vi "Get Property Enum Values.vi"(0 "SLSC Remote in":refnum<class "SLSC Remote.lvclass">, 5 "property":refnum<k21>, 11 "error in (no error)":errorcluster) -> (4 "SLSC Remote out":refnum<class "SLSC Remote.lvclass">, 6 "property out":refnum<k21>, 10 "Prop.Enum.Values":i32[](array[numeric]), 15 "error out":errorcluster)   [LabVIEW 2016, in "SLSC Interfaces.lvlib" / "SLSC Remote.lvclass"]
uses:
  SLSC Remote.lvclass
  C:/Users/tblair/Documents/Git Projects/SLSC-Interface/Source/SLSC Interface Class/SLSC Interface.lvclass
  <vilib>/National Instruments/JSON Support for LabVIEW/JSON Data Classes/JSON Object/JSON Object.lvclass
  C:/Program Files (x86)/National Instruments/LabVIEW 2016/vi.lib/National Instruments/JSON Support for LabVIEW/JSON Data Classes/JSON Datatype/JSON Datatype.lvclass
  <vilib>/National Instruments/JSON Support for LabVIEW/JSON Data Classes/JSON Object/New JSON Object (Empty).vi
  <vilib>/National Instruments/JSON Support for LabVIEW/JSON Data Classes/JSON Object/Insert Key Value Pair (Single String).vi
  <vilib>/NI/NI JSONRPC Server Framework/Classes/Server/Format Client Request (Auto-Increment).vi
  <vilib>/httpClient/POSTBuffer.vi
  <vilib>/National Instruments/JSON Support for LabVIEW/JSON Data Classes/JSON Datatype/To More Specific Type (Object).vi
  <vilib>/National Instruments/JSON Support for LabVIEW/JSON Data Classes/JSON Object/Get Value (Array).vi
  <vilib>/National Instruments/JSON Support for LabVIEW/JSON Data Classes/JSON Array/Index Array (Numeric Value).vi
  <vilib>/NI/NI JSONRPC Server Framework/Classes/Server/JSONRPC Server.lvclass
  <vilib>/httpClient/LabVIEWHTTPClient.lvlib
  <vilib>/National Instruments/JSON Support for LabVIEW/JSON Data Classes/JSON Datatype/JSON Datatype.lvclass
  <vilib>/National Instruments/JSON Support for LabVIEW/JSON Data Classes/JSON Array/JSON Array.lvclass
  C:/Program Files (x86)/National Instruments/LabVIEW 2016/vi.lib/National Instruments/JSON Support for LabVIEW/JSON Data Classes/JSON Structured Type/JSON Structured Type.lvclass
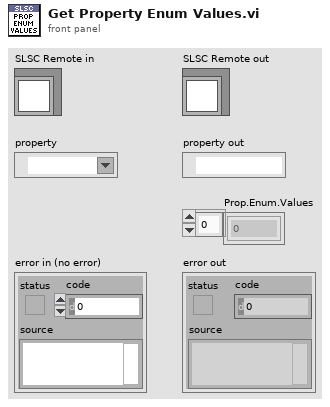
[diagram p1: front panel]
types:
  T1 = typedef "LabVIEWHTTPClient.lvlib/ClientHandle.ctl" = refnum<k1>
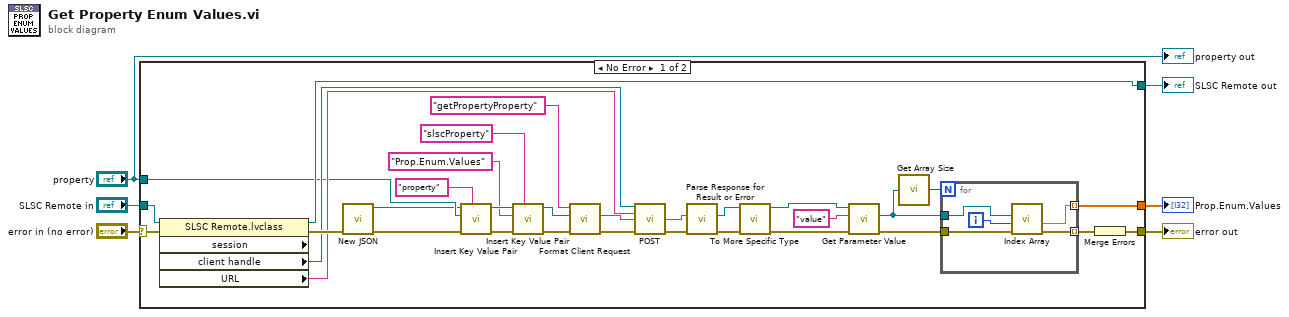
[diagram p0: block diagram]
diagram:
  n1 = case shown="No Error" "error in (no error)" {
    selector: "error in (no error)" -> [w36 w44]
    tunnel: "SLSC Remote in" -> [w38 w45]
    tunnel: [w37 w45] -> w4
    tunnel: [w13 w44] -> w2
    tunnel: "property" -> [w12 _]
    tunnel: [w14 _] -> w1
    frame No Error {
      n2 = property class="SLSC Remote.lvclass" props=["session", "client handle", "URL"](reference=w38, error in=w36) -> (reference out=w37:refnum<class "SLSC Remote.lvclass">, error out=w35:errorcluster, "client handle"=w31:T1, "URL"=w30:string)  [unwired: 1 out]
      n3 = call-poly <vilib>:"New JSON.vi"("error in (no error)"=w35) -> ("error out"=w34:errorcluster, "JSON Object out"=w9:refnum<class "JSON Object.lvclass">)  [unwired: 9 in]
      n4 = call-poly <vilib>:"Insert Key Value Pair.vi"("key"="property" ("Name"), "error in (no error)"=w34, "value"=w12, "JSON Object in"=w9) -> ("error out"=w24:errorcluster, "JSON Object out"=w10:refnum<class "JSON Object.lvclass">)  [unwired: 5 in, 1 out]
      n5 = call-poly <vilib>:"Insert Key Value Pair.vi"("key"="slscProperty" ("Name"), "error in (no error)"=w24, "value"="Prop.Enum.Values" ("String"), "JSON Object in"=w10) -> ("error out"=w25:errorcluster, "JSON Object out"=w26:refnum<class "JSON Object.lvclass">)  [unwired: 5 in, 1 out]
      n6 = call-poly <vilib>:"Format Client Request.vi"("error in (no error)"=w25, "JSON in"=w26, "method"="getPropertyProperty") -> ("error out"=w29:errorcluster, "Request String"=w32:string)  [unwired: 7 in]
      n7 = call-poly <vilib>:"POST.vi"("client handle"=w31, "url"=w30, "buffer"=w32, "error in (no error)"=w29) -> ("body"=w28:string, "error out"=w27:errorcluster)  [unwired: 8 in, 2 out]
      n8 = call <vilib>:"Parse Response for Result or Error.vi"("error in"=w27, "Response String In"=w28) -> ("error out"=w16:errorcluster, "JSON out"=w17:refnum<class "JSON Datatype.lvclass">)  [unwired: 7 in, 1 out]
      n9 = call-poly <vilib>:"To More Specific Type.vi"("error in (no error)"=w16, "JSON Datatype in"=w17) -> ("error out"=w23:errorcluster, "JSON Datatype out"=w22:refnum<class "JSON Object.lvclass">)  [unwired: 8 in]
      n10 = call-poly <vilib>:"Get Parameter Value.vi"("error in (no error)"=w23, "key"="value" ("Parameter Name"), "JSON Object in"=w22) -> ("error out"=w19:errorcluster, "value"=w20:refnum<class "JSON Array.lvclass">)  [unwired: 6 in, 1 out]
      n11 = call <vilib>:"Get Array Size.vi"("JSON Array in"=w20) -> ("size(s)"=w21:i32)
      n12 = for {
        N: w21 -> [_]
        tunnel: w20 -> [w42]
        tunnel: w19 -> [w41]
        tunnel: [w40] -> w18 mode=indexing
        tunnel: [w39] -> w14 mode=indexing
        i -> [w43]
        n13 = call-poly <vilib>:"Index Array.vi"("error in (no error)"=w41, "index"=w43, "JSON Array in"=w42) -> ("error out"=w40:errorcluster, "Numeric"=w39:dbl)  [unwired: 7 in]
      }
      n14 = Merge Errors(w18) -> (w13:errorcluster)
    }
    frame Error {
    }
  }
  "error out" <- w2
  "SLSC Remote out" <- w4
  "Prop.Enum.Values" <- w1
  "property out" <- "property"
